vi "OpenArm.vi"(7 "Wrist PID":T1={"No Bin"={"P"=30.0, "I"=0.0, "D"=100.0}, "Bin"={"P"=0.0, "I"=0.0, "D"=0.0}}, 8 "error in (no error)":errorcluster, 10 "Pivot PID":T1={"No Bin"={"P"=30.0, "I"=0.0, "D"=20.0}, "Bin"={"P"=0.0, "I"=0.0, "D"=0.0}}, 11 "Extension PID":T1={"No Bin"={"P"=40.0, "I"=0.0, "D"=0.0}, "Bin"={"P"=0.0, "I"=0.0, "D"=0.0}}) -> (0 "error out":errorcluster)   [LabVIEW 2014]
uses:
  <vilib>/Rock Robotics/WPI/CAN/TalonSRX/WPI_CANTalonSRX_APIControlMode.ctl
  <vilib>/Rock Robotics/WPI/CAN/TalonSRX/WPI_CANTalonSRX_APIFeedbackSelect.ctl
  Robot Global Data.vi
  <vilib>/Rock Robotics/WPI/MotorControl/WPI_MotorControlOpenCANTalonSRX.vi
panel:
  in  "Reverse Pivot Limit":dbl=-512.0
  in  "Forward Pivot Limit":dbl
  in  "Reverse Claw Limit":dbl=64.0 format="%#_13g"
  in  "Forward Claw Limit":dbl=215.0 format="%#_13g"
  in  "Forward Wrist Limit":dbl=256.0
  in  "Reverse Wrist Limit":dbl=-256.0
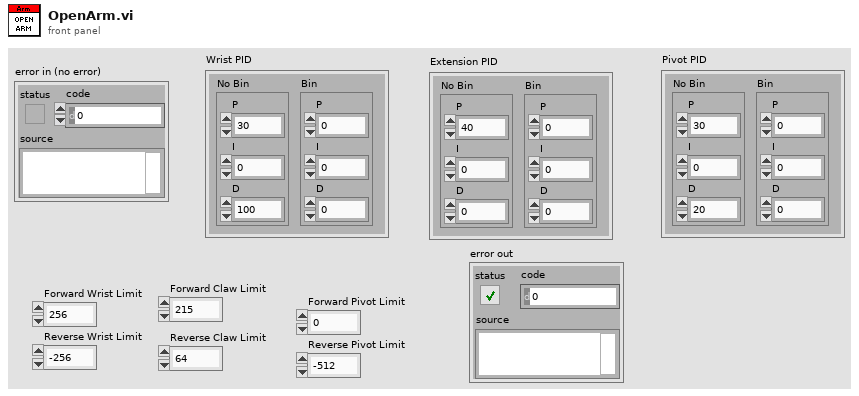
[diagram p1: front panel]
types:
  T1 = cluster{"No Bin":cluster{"P":dbl, "I":dbl, "D":dbl}, "Bin":cluster{"P":dbl, "I":dbl, "D":dbl}}
  T2 = typedef "WPI_CANTalonSRX_APIControlMode.ctl" = enum8{"Percent VBus", "Speed", "Position", "Slave", "Unchanged / Invalid"}
  T3 = typedef "WPI_CANTalonSRX_APIFeedbackSelect.ctl" = enum16{"Digital Quadrature Encoder", "Analog Potentiometer", "Analog Encoder"}
  T4 = typedef "WPI_MotorControlDeviceRef.ctl" = cluster{"DeviceStatus":errorcluster, "Type":T5, "PWM":cluster{"Controller":T6, "PWM Channel":T7, "DeadBand":T8}, "CAN":cluster{"Device Number":u8, "Control Mode":T9, "Semaphore":T10, "Max Vout":dbl, "TalonSRX Control Mode":T2}, "Invert":bool, "TransformRef":T11, "InvTransformRef":T11}
  T5 = typedef "WPI_MotorControlType.ctl" = enum16{"PWM", "CAN", "CANTalonSRX"}
  T6 = typedef "FPGA_TypedefDigitalModule.ctl" = enum16{"Controller 1"}
  T7 = typedef "FPGA_DIOPWMChannel.ctl" = enum8{"PWM 0", "PWM 1", "PWM 2", "PWM 3", "PWM 4", "PWM 5", "PWM 6", "PWM 7", "PWM 8", "PWM 9", "PWM MXP 0", "PWM MXP 1", "PWM MXP 2", "PWM MXP 3", "PWM MXP 4", "PWM MXP 5", "PWM MXP 6", "PWM MXP 7", "PWM MXP 8", "PWM MXP 9", "Invalid"}
  T8 = typedef "WPI_PWMDeadband.ctl" = cluster{"Name":string, "maxPositivePwm":i32, "minPositivePwm":i32, "centerPwm":i32, "maxNegativePwm":i32, "minNegativePwm":i32, "angularRange":u16}
  T9 = typedef "WPI_CANJaguar_ControlMode.ctl" = enum8{"Percent VBus", "Current", "Speed", "Position", "Voltage"}
  T10 = typedef "Semaphore RefNum" = refnum<k1>
  T11 = typedef "WPI_PWMTransform_ConPane.ctl" = refnum<vi>
  T12 = typedef "WPI_CANTalonSRX_GlobalStatus.ctl" = cluster{"Applied Throttle":dbl, "Module Enabled":bool, "CAN Error":errorcluster, "Closed Loop Error":dbl, "Forward Limit Switch Closed":bool, "Reverse Limit Switch Closed":bool, "Sensor Position":dbl, "Sensor Velocity":dbl, "Current":dbl, "Sticky Fault - Over Temp":bool, "Sticky Fault - Under Voltage":bool, "Sticky Fault - Forward Limit":bool, "Sticky Fault - Reverse Limit":bool, "Sticky Fault - Forward Soft Limit":bool, "Sticky Fault - Reverse Soft Limit":bool, "Brake is Enabled":bool, "Encoder Position":dbl, "Encoder Velocity":dbl, "Encoder Index Count":dbl, "Encoder A Pin State":bool, "Encoder B Pin State":bool, "Encoder Index Pin State":bool, "Analog In":dbl, "Analog In Velocity":dbl, "Temperature (C)":dbl, "Battery Voltage":dbl}
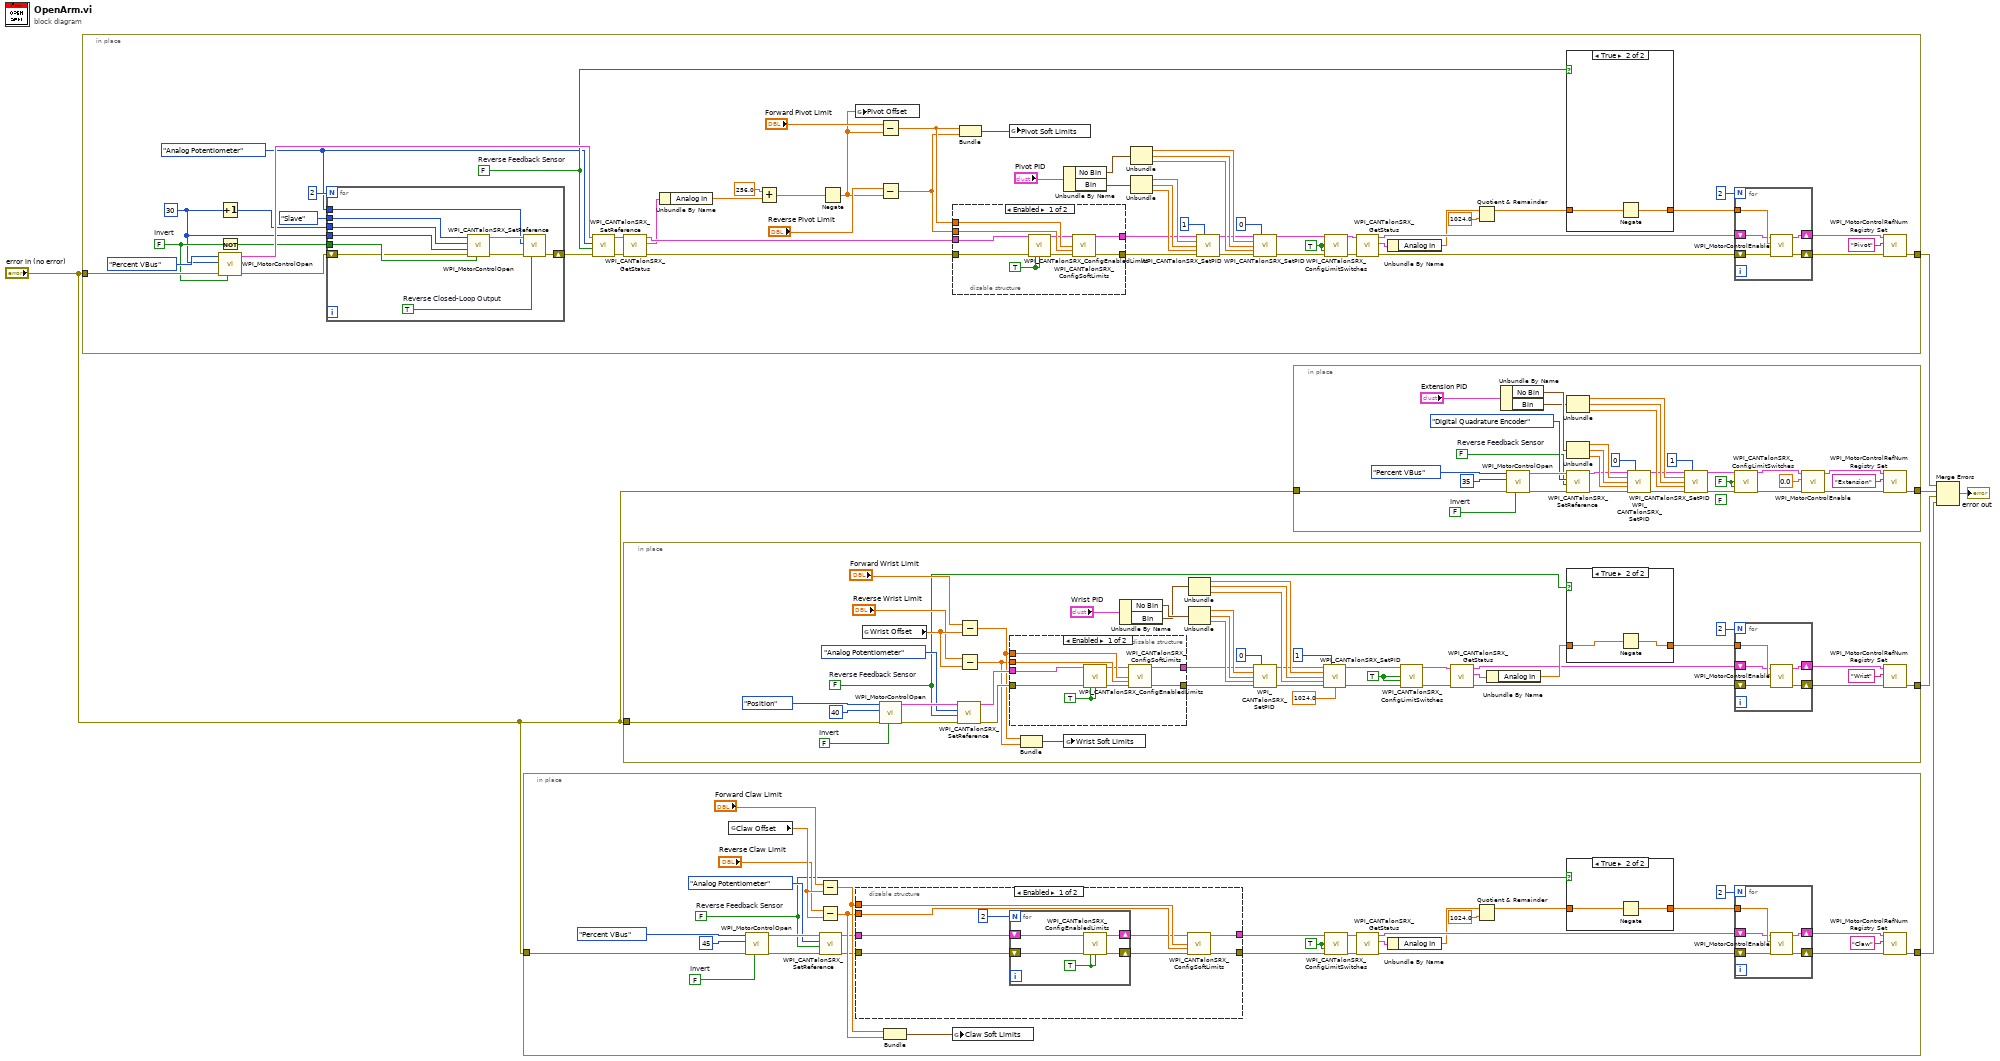
[diagram p0: block diagram]
diagram:
  n1 = in-place {
    in-place-border: [w62] -> w6
    in-place-border: "error in (no error)" -> [w61]
    w47 = FALSE  # Reverse Feedback Sensor
    w36 = FALSE  # Invert
    w59 = TRUE ("Forward Limit Switch Normally Open")
    w31 = WPI_CANTalonSRX_APIFeedbackSelect."Analog Potentiometer" ("Feedback Reference")
    w35 = u8 30 ("Pivot ID")
    n2 = Increment(x=w35) -> (x+1=w38:u8)
    n3 = Not(x=w36) -> (.not. x?=w37:bool)
    n4 = call-poly <vilib>:"WPI_MotorControlOpen.vi"("Invert"=w36, "error in (no error)"=w61, "Device Number"=w35, "Control Mode"=WPI_CANTalonSRX_APIControlMode."Percent VBus") -> ("error out"=w34:errorcluster, "MotorControlDeviceRef"=w60:T4)  [unwired: 6 in]
    n5 = for {
      N: 2 -> [_]
      tunnel: WPI_CANTalonSRX_APIControlMode."Slave" ("Control Mode") -> [w75]
      tunnel: w38 -> [w74]
      tunnel: w37 -> [w73]
      tunnel: w35 -> [w72]
      shift-right: [w68] -> w33
      shift-left: w34 -> [w71]
      tunnel: w31 -> [w67]
      w66 = TRUE  # Reverse Closed-Loop Output
      n6 = call-poly <vilib>:"WPI_MotorControlOpen.vi"("Invert"=w73, "error in (no error)"=w71, "Master Device Number"=w72, "Device Number"=w74, "Control Mode"=w75) -> ("error out"=w69:errorcluster, "MotorControlDeviceRef"=w70:T4)  [unwired: 5 in]
      n7 = call <vilib>:"WPI_CANTalonSRX_SetReference.vi"("Reverse Closed-Loop Output"=w66, "error in (no error)"=w69, "Feedback Reference"=w67, "CAN Talon SRX Ref"=w70) -> ("error out"=w68:errorcluster)  [unwired: 6 in, 1 out]
    }
    n8 = call <vilib>:"WPI_CANTalonSRX_SetReference.vi"("error in (no error)"=w33, "Reverse Feedback Sensor"=w47, "Feedback Reference"=w31, "CAN Talon SRX Ref"=w60) -> ("error out"=w14:errorcluster, "CAN Talon SRX Ref Out"=w15:T4)  [unwired: 6 in]
    n9 = call <vilib>:"WPI_CANTalonSRX_GetStatus.vi"("error in (no error)"=w14, "CAN Talon SRX Ref"=w15) -> ("error out"=w13:errorcluster, "Talon SRX Status"=w11:T12, "CAN Talon SRX Ref Out"=w12:T4)  [unwired: 7 in]
    n10 = Unbundle By Name(w11) -> ("Analog In"=w9:dbl)
    n11 = Add(x=256.0, y=w9) -> (x+y=w8:dbl)
    n12 = Negate(x=w8) -> (-x=w7:dbl)
    n13 = global write "Robot Global Data.vi" "Pivot Offset"(w7) -> ()
    n14 = Subtract(x="Forward Pivot Limit", y=w7) -> (x-y=w54:dbl)
    n15 = Subtract(x="Reverse Pivot Limit", y=w7) -> (x-y=w53:dbl)
    n16 = disable-structure shown="Enabled" {
      disable-tunnel: w12 -> [w80 w86]
      disable-tunnel: w13 -> [w81 w85]
      disable-tunnel: w54 -> [w84 _]
      disable-tunnel: w53 -> [w83 _]
      disable-tunnel: [w78 w85] -> w49
      disable-tunnel: [w76 w86] -> w48
      frame Enabled {
        w82 = TRUE ("Forward Soft Limit Enable")
        n17 = call <vilib>:"WPI_CANTalonSRX_ConfigEnabledLimits.vi"("CAN Talon SRX Ref"=w80, "error in (no error)"=w81, "Forward Soft Limit Enable"=w82, "Reverse Soft Limit Enable"=w82) -> ("CAN Talon SRX Ref Out"=w77:T4, "error out"=w79:errorcluster)  [unwired: 10 in]
        n18 = call <vilib>:"WPI_CANTalonSRX_ConfigSoftLimits.vi"("CAN Talon SRX Ref"=w77, "Forward Limit Position"=w84, "Reverse Limit Position"=w83, "error in (no error)"=w79) -> ("CAN Talon SRX Ref Out"=w76:T4, "error out"=w78:errorcluster)  [unwired: 10 in]
      }
      frame Disabled {
      }
    }
    n19 = Bundle(w54, w53) -> (w55:cluster{dbl, dbl})  [unwired: 1 in]
    n20 = global write "Robot Global Data.vi" "Pivot Soft Limits"(w55) -> ()
    n21 = Unbundle By Name("Pivot PID") -> ("No Bin"=w20:cluster{"P":dbl, "I":dbl, "D":dbl}, "Bin"=w19:cluster{"P":dbl, "I":dbl, "D":dbl})
    n22 = Unbundle(w20) -> ("P"=w25:dbl, "I"=w26:dbl, "D"=w27:dbl)
    n23 = Unbundle(w19) -> ("P"=w63:dbl, "I"=w64:dbl, "D"=w65:dbl)
    n24 = call <vilib>:"WPI_CANTalonSRX_SetPID.vi"("CAN Talon SRX Ref"=w48, "Parameter Slot"=u8 1, "P"=w63, "I"=w64, "D"=w65, "error in (no error)"=w49) -> ("CAN Talon SRX Ref Out"=w23:T4, "error out"=w22:errorcluster)  [unwired: 8 in]
    n25 = call <vilib>:"WPI_CANTalonSRX_SetPID.vi"("CAN Talon SRX Ref"=w23, "Parameter Slot"=u8 0, "P"=w25, "I"=w26, "D"=w27, "error in (no error)"=w22) -> ("CAN Talon SRX Ref Out"=w18:T4, "error out"=w17:errorcluster)  [unwired: 8 in]
    n26 = call <vilib>:"WPI_CANTalonSRX_ConfigLimitSwitches.vi"("CAN Talon SRX Ref"=w18, "Forward Limit Switch Normally Open"=w59, "Reverse Limit Switch Normally Open"=w59, "error in (no error)"=w17) -> ("CAN Talon SRX Ref Out"=w51:T4, "error out"=w52:errorcluster)  [unwired: 10 in]
    n27 = call <vilib>:"WPI_CANTalonSRX_GetStatus.vi"("error in (no error)"=w52, "CAN Talon SRX Ref"=w51) -> ("error out"=w44:errorcluster, "Talon SRX Status"=w50:T12, "CAN Talon SRX Ref Out"=w45:T4)  [unwired: 7 in]
    n28 = Unbundle By Name(w50) -> ("Analog In"=w29:dbl)
    n29 = Quotient & Remainder(x=w29, y=1024.0) -> (x-y*floor(x/y)=w30:dbl)  [unwired: 1 out]
    n30 = case shown="True" w47 {
      tunnel: w30 -> [w92 w94]
      tunnel: [w92 w93] -> w46
      frame False {
      }
      frame True {
        n31 = Negate(x=w94) -> (-x=w93:dbl)
      }
    }
    n32 = for {
      N: 2 -> [_]
      tunnel: w46 -> [w91]
      shift-right: [w87] -> w42
      shift-left: w45 -> [w90]
      shift-right: [w88] -> w43
      shift-left: w44 -> [w89]
      n33 = call <vilib>:"WPI_MotorControlEnable.vi"("error in (no error)"=w89, "Encoder Initial Position"=w91, "CAN Jaguar Ref"=w90) -> ("error out"=w88:errorcluster, "CAN Jaguar Ref Out"=w87:T4)  [unwired: 7 in]
    }
    n34 = call <vilib>:"WPI_MotorControlRefNum Registry Set.vi"("error in (no error)"=w43, "refnum name"="Pivot", "MotorControlDevRef"=w42) -> ("error out"=w62:errorcluster)  [unwired: 7 in, 1 out]
  }
  n35 = in-place {
    in-place-border: [w123] -> w2
    in-place-border: "error in (no error)" -> [w122]
    w98 = FALSE  # Reverse Feedback Sensor
    w118 = TRUE ("Forward Limit Switch Normally Open")
    w124 = FALSE  # Invert
    n36 = global read "Robot Global Data.vi" "Claw Offset"() -> (w119:dbl)
    n37 = call-poly <vilib>:"WPI_MotorControlOpen.vi"("Invert"=w124, "error in (no error)"=w122, "Device Number"=u8 45 ("Claw ID"), "Control Mode"=WPI_CANTalonSRX_APIControlMode."Percent VBus") -> ("error out"=w112:errorcluster, "MotorControlDeviceRef"=w121:T4)  [unwired: 6 in]
    n38 = Subtract(x="Forward Claw Limit", y=w119) -> (x-y=w114:dbl)
    n39 = Subtract(x="Reverse Claw Limit", y=w119) -> (x-y=w113:dbl)
    n40 = call <vilib>:"WPI_CANTalonSRX_SetReference.vi"("error in (no error)"=w112, "Reverse Feedback Sensor"=w98, "Feedback Reference"=WPI_CANTalonSRX_APIFeedbackSelect."Analog Potentiometer", "CAN Talon SRX Ref"=w121) -> ("error out"=w99:errorcluster, "CAN Talon SRX Ref Out"=w100:T4)  [unwired: 6 in]
    n41 = disable-structure shown="Enabled" {
      disable-tunnel: w114 -> [w136 _]
      disable-tunnel: w113 -> [w135 _]
      disable-tunnel: [w134 w142] -> w102
      disable-tunnel: [w133 w143] -> w101
      disable-tunnel: w100 -> [w132 w143]
      disable-tunnel: w99 -> [w131 w142]
      frame Enabled {
        n42 = for {
          N: 2 -> [_]
          shift-right: [w138] -> w130
          shift-left: w132 -> [w140]
          shift-right: [w137] -> w129
          shift-left: w131 -> [w139]
          w141 = TRUE ("Forward Soft Limit Enable")
          n43 = call <vilib>:"WPI_CANTalonSRX_ConfigEnabledLimits.vi"("CAN Talon SRX Ref"=w140, "error in (no error)"=w139, "Forward Soft Limit Enable"=w141, "Reverse Soft Limit Enable"=w141) -> ("CAN Talon SRX Ref Out"=w138:T4, "error out"=w137:errorcluster)  [unwired: 10 in]
        }
        n44 = call <vilib>:"WPI_CANTalonSRX_ConfigSoftLimits.vi"("CAN Talon SRX Ref"=w130, "Forward Limit Position"=w136, "Reverse Limit Position"=w135, "error in (no error)"=w129) -> ("CAN Talon SRX Ref Out"=w133:T4, "error out"=w134:errorcluster)  [unwired: 10 in]
      }
      frame Disabled {
      }
    }
    n45 = Bundle(w114, w113) -> (w115:cluster{dbl, dbl})  [unwired: 1 in]
    n46 = global write "Robot Global Data.vi" "Claw Soft Limits"(w115) -> ()
    n47 = call <vilib>:"WPI_CANTalonSRX_ConfigLimitSwitches.vi"("CAN Talon SRX Ref"=w101, "Forward Limit Switch Normally Open"=w118, "Reverse Limit Switch Normally Open"=w118, "error in (no error)"=w102) -> ("CAN Talon SRX Ref Out"=w106:T4, "error out"=w105:errorcluster)  [unwired: 10 in]
    n48 = call <vilib>:"WPI_CANTalonSRX_GetStatus.vi"("error in (no error)"=w105, "CAN Talon SRX Ref"=w106) -> ("error out"=w108:errorcluster, "Talon SRX Status"=w111:T12, "CAN Talon SRX Ref Out"=w109:T4)  [unwired: 7 in]
    n49 = Unbundle By Name(w111) -> ("Analog In"=w97:dbl)
    n50 = Quotient & Remainder(x=w97, y=1024.0) -> (x-y*floor(x/y)=w96:dbl)  [unwired: 1 out]
    n51 = case shown="True" w98 {
      tunnel: w96 -> [w149 w151]
      tunnel: [w149 w150] -> w110
      frame False {
      }
      frame True {
        n52 = Negate(x=w151) -> (-x=w150:dbl)
      }
    }
    n53 = for {
      N: 2 -> [_]
      tunnel: w110 -> [w148]
      shift-right: [w144] -> w104
      shift-left: w109 -> [w147]
      shift-right: [w145] -> w103
      shift-left: w108 -> [w146]
      n54 = call <vilib>:"WPI_MotorControlEnable.vi"("error in (no error)"=w146, "Encoder Initial Position"=w148, "CAN Jaguar Ref"=w147) -> ("error out"=w145:errorcluster, "CAN Jaguar Ref Out"=w144:T4)  [unwired: 7 in]
    }
    n55 = call <vilib>:"WPI_MotorControlRefNum Registry Set.vi"("error in (no error)"=w103, "refnum name"="Claw", "MotorControlDevRef"=w104) -> ("error out"=w123:errorcluster)  [unwired: 7 in, 1 out]
  }
  n56 = in-place {
    in-place-border: [w192] -> w4
    in-place-border: "error in (no error)" -> [w191]
    w165 = FALSE  # Reverse Feedback Sensor
    w183 = TRUE ("Forward Limit Switch Normally Open")
    w193 = FALSE  # Invert
    n57 = global read "Robot Global Data.vi" "Wrist Offset"() -> (w184:dbl)
    n58 = call-poly <vilib>:"WPI_MotorControlOpen.vi"("Invert"=w193, "error in (no error)"=w191, "Device Number"=u8 40 ("Wrist ID"), "Control Mode"=WPI_CANTalonSRX_APIControlMode."Position") -> ("error out"=w189:errorcluster, "MotorControlDeviceRef"=w190:T4)  [unwired: 6 in]
    n59 = call <vilib>:"WPI_CANTalonSRX_SetReference.vi"("error in (no error)"=w189, "Reverse Feedback Sensor"=w165, "Feedback Reference"=WPI_CANTalonSRX_APIFeedbackSelect."Analog Potentiometer", "CAN Talon SRX Ref"=w190) -> ("error out"=w186:errorcluster, "CAN Talon SRX Ref Out"=w185:T4)  [unwired: 6 in]
    n60 = Subtract(x="Forward Wrist Limit", y=w184) -> (x-y=w181:dbl)
    n61 = Subtract(x="Reverse Wrist Limit", y=w184) -> (x-y=w180:dbl)
    n62 = disable-structure shown="Enabled" {
      disable-tunnel: w186 -> [w200 w208]
      disable-tunnel: w185 -> [w199 w209]
      disable-tunnel: w181 -> [w207 _]
      disable-tunnel: w180 -> [w206 _]
      disable-tunnel: [w203 w209] -> w179
      disable-tunnel: [w204 w208] -> w178
      frame Enabled {
        w205 = TRUE ("Forward Soft Limit Enable")
        n63 = call <vilib>:"WPI_CANTalonSRX_ConfigEnabledLimits.vi"("CAN Talon SRX Ref"=w199, "error in (no error)"=w200, "Forward Soft Limit Enable"=w205, "Reverse Soft Limit Enable"=w205) -> ("CAN Talon SRX Ref Out"=w202:T4, "error out"=w201:errorcluster)  [unwired: 10 in]
        n64 = call <vilib>:"WPI_CANTalonSRX_ConfigSoftLimits.vi"("CAN Talon SRX Ref"=w202, "Forward Limit Position"=w207, "Reverse Limit Position"=w206, "error in (no error)"=w201) -> ("CAN Talon SRX Ref Out"=w203:T4, "error out"=w204:errorcluster)  [unwired: 10 in]
      }
      frame Disabled {
      }
    }
    n65 = Bundle(w181, w180) -> (w182:cluster{dbl, dbl})  [unwired: 1 in]
    n66 = global write "Robot Global Data.vi" "Wrist Soft Limits"(w182) -> ()
    n67 = Unbundle By Name("Wrist PID") -> ("No Bin"=w154:cluster{"P":dbl, "I":dbl, "D":dbl}, "Bin"=w153:cluster{"P":dbl, "I":dbl, "D":dbl})
    n68 = Unbundle(w153) -> ("P"=w161:dbl, "I"=w162:dbl, "D"=w163:dbl)
    n69 = Unbundle(w154) -> ("P"=w194:dbl, "I"=w195:dbl, "D"=w196:dbl)
    n70 = call <vilib>:"WPI_CANTalonSRX_SetPID.vi"("CAN Talon SRX Ref"=w179, "Parameter Slot"=u8 0, "P"=w194, "I"=w195, "D"=w196, "error in (no error)"=w178) -> ("CAN Talon SRX Ref Out"=w159:T4, "error out"=w158:errorcluster)  [unwired: 8 in]
    n71 = call <vilib>:"WPI_CANTalonSRX_SetPID.vi"("CAN Talon SRX Ref"=w159, "Parameter Slot"=u8 1, "P"=w161, "I"=w162, "D"=w163, "error in (no error)"=w158, "I Zone"=1024.0) -> ("CAN Talon SRX Ref Out"=w157:T4, "error out"=w156:errorcluster)  [unwired: 7 in]
    n72 = call <vilib>:"WPI_CANTalonSRX_ConfigLimitSwitches.vi"("CAN Talon SRX Ref"=w157, "Forward Limit Switch Normally Open"=w183, "Reverse Limit Switch Normally Open"=w183, "error in (no error)"=w156) -> ("CAN Talon SRX Ref Out"=w171:T4, "error out"=w170:errorcluster)  [unwired: 10 in]
    n73 = call <vilib>:"WPI_CANTalonSRX_GetStatus.vi"("error in (no error)"=w170, "CAN Talon SRX Ref"=w171) -> ("error out"=w173:errorcluster, "Talon SRX Status"=w177:T12, "CAN Talon SRX Ref Out"=w174:T4)  [unwired: 7 in]
    n74 = Unbundle By Name(w177) -> ("Analog In"=w176:dbl)
    n75 = case shown="True" w165 {
      tunnel: w176 -> [w215 w217]
      tunnel: [w215 w216] -> w175
      frame False {
      }
      frame True {
        n76 = Negate(x=w217) -> (-x=w216:dbl)
      }
    }
    n77 = for {
      N: 2 -> [_]
      tunnel: w175 -> [w214]
      shift-right: [w210] -> w169
      shift-left: w174 -> [w213]
      shift-right: [w211] -> w168
      shift-left: w173 -> [w212]
      n78 = call <vilib>:"WPI_MotorControlEnable.vi"("error in (no error)"=w212, "Encoder Initial Position"=w214, "CAN Jaguar Ref"=w213) -> ("error out"=w211:errorcluster, "CAN Jaguar Ref Out"=w210:T4)  [unwired: 7 in]
    }
    n79 = call <vilib>:"WPI_MotorControlRefNum Registry Set.vi"("error in (no error)"=w168, "refnum name"="Wrist", "MotorControlDevRef"=w169) -> ("error out"=w192:errorcluster)  [unwired: 7 in, 1 out]
  }
  n80 = in-place {
    in-place-border: [w246] -> w5
    in-place-border: "error in (no error)" -> [w245]
    (unwired) FALSE ("Forward Limit Switch Normally Open")
    w235 = FALSE  # Reverse Feedback Sensor
    w236 = FALSE ("Forward Limit Switch Normally Open")
    w237 = FALSE  # Invert
    n81 = Unbundle By Name("Extension PID") -> ("No Bin"=w228:cluster{"P":dbl, "I":dbl, "D":dbl}, "Bin"=w218:cluster{"P":dbl, "I":dbl, "D":dbl})
    n82 = call-poly <vilib>:"WPI_MotorControlOpen.vi"("Invert"=w237, "error in (no error)"=w245, "Device Number"=u8 35 ("Extension ID"), "Control Mode"=WPI_CANTalonSRX_APIControlMode."Percent VBus") -> ("error out"=w240:errorcluster, "MotorControlDeviceRef"=w243:T4)  [unwired: 6 in]
    n83 = Unbundle(w218) -> ("P"=w224:dbl, "I"=w225:dbl, "D"=w226:dbl)
    n84 = Unbundle(w228) -> ("P"=w247:dbl, "I"=w248:dbl, "D"=w249:dbl)
    n85 = call <vilib>:"WPI_CANTalonSRX_SetReference.vi"("error in (no error)"=w240, "Reverse Feedback Sensor"=w235, "Feedback Reference"=WPI_CANTalonSRX_APIFeedbackSelect."Digital Quadrature Encoder", "CAN Talon SRX Ref"=w243) -> ("error out"=w241:errorcluster, "CAN Talon SRX Ref Out"=w242:T4)  [unwired: 6 in]
    n86 = call <vilib>:"WPI_CANTalonSRX_SetPID.vi"("CAN Talon SRX Ref"=w242, "Parameter Slot"=u8 0, "P"=w247, "I"=w248, "D"=w249, "error in (no error)"=w241) -> ("CAN Talon SRX Ref Out"=w222:T4, "error out"=w221:errorcluster)  [unwired: 8 in]
    n87 = call <vilib>:"WPI_CANTalonSRX_SetPID.vi"("CAN Talon SRX Ref"=w222, "Parameter Slot"=u8 1, "P"=w224, "I"=w225, "D"=w226, "error in (no error)"=w221) -> ("CAN Talon SRX Ref Out"=w220:T4, "error out"=w219:errorcluster)  [unwired: 8 in]
    n88 = call <vilib>:"WPI_CANTalonSRX_ConfigLimitSwitches.vi"("CAN Talon SRX Ref"=w220, "Forward Limit Switch Normally Open"=w236, "Reverse Limit Switch Normally Open"=w236, "error in (no error)"=w219) -> ("CAN Talon SRX Ref Out"=w230:T4, "error out"=w231:errorcluster)  [unwired: 10 in]
    n89 = call <vilib>:"WPI_MotorControlEnable.vi"("error in (no error)"=w231, "Encoder Initial Position"=0.0 ("Analog In"), "CAN Jaguar Ref"=w230) -> ("error out"=w233:errorcluster, "CAN Jaguar Ref Out"=w234:T4)  [unwired: 7 in]
    n90 = call <vilib>:"WPI_MotorControlRefNum Registry Set.vi"("error in (no error)"=w233, "refnum name"="Extension", "MotorControlDevRef"=w234) -> ("error out"=w246:errorcluster)  [unwired: 7 in, 1 out]
  }
  n91 = Merge Errors(w6, w5, w4, w2) -> (→"error out":errorcluster)
